vi "Convert State For Save.vi"(2 "Container State":T1, 3 "Display State":T2) -> (1 "Display State To Save":variant)   [LabVIEW 2017, in "3D Bar.xctl"]
uses:
  <vilib>/Math Plots/3D Math Plots/3D Bar/3D Bar XCtrl/3D Bar.xctl
  <vilib>/Math Plots/3D Math Plots/3D Bar/3D Bar XCtrl/State.ctl
  <vilib>/Math Plots/3D Math Plots/3D Bar/3D Bar/3D Bar.lvclass
  e:/builds/penguin/labview/branches/2017/dev/dist/vi.lib/Math Plots/3D Math Plots/3D Plot/3D Plot/3D Plot.lvclass
  <vilib>/Math Plots/3D Math Plots/3D Plot/Action String/3DMathPlot Ctrl Act Queue.ctl
  <vilib>/Math Plots/3D Math Plots/3D Plot/Action String/3DMathPlot Ctrl Act Cluster.ctl
  <vilib>/Math Plots/3D Math Plots/3D Plot/Action String/3DMathPlot State Class.ctl
  <vilib>/_xctls/Container State.ctl
  <vilib>/Math Plots/3D Math Plots/3D Plot/3D Plot/3D Plot.lvclass
  <vilib>/_xctls/XControlSupport.lvlib
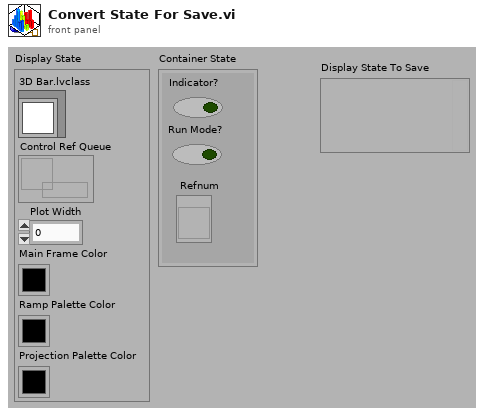
[diagram p1: front panel]
types:
  T1 = typedef "XControlSupport.lvlib/Container State.ctl" = cluster{"Indicator?":bool, "Run Mode?":bool, " Refnum":refnum<vi>}
  T2 = typedef "3D Bar.xctl/State.ctl" = cluster{"3D Bar.lvclass":refnum<class "3D Bar.lvclass">, "Control Ref Queue":T3, "Plot Width":u32, "Main Frame Color":u32, "Ramp Palette Color":u32, "Projection Palette Color":u32}
  T3 = typedef "3DMathPlot Ctrl Act Queue.ctl" = refnum<queue>
  T4 = enum32{"Towards X-Y Plane", "Towards X-Z Plane", "Towards Y-Z Plane", "User Defined"}
  T5 = typedef "3DMathPlot Ctrl Act Cluster.ctl" = cluster{"3D Picture Control":refnum<vi>, "Render Window Refnum":refnum<vi>, "XY Graph":refnum<vi>, "Intensity Graph":refnum<vi>, "Color Legend Palette":refnum<vi>, "Projection Palette":refnum<vi>, "XControl  Ref":refnum<vi>, "Facade Ref":refnum<vi>, "Export Image Ref":refnum<vi>, "Clear Data Flag":bool, "Display State Change Class":T6}
  T6 = typedef "3DMathPlot State Class.ctl" = enum16{"Update All Objects (Undo)", "Update Light Object Only", "Update Axis Object Only", "Update Plot Object Only", "Update Cursor Object Only", "Update Axis Plot Cursor Objects", "No Update"}
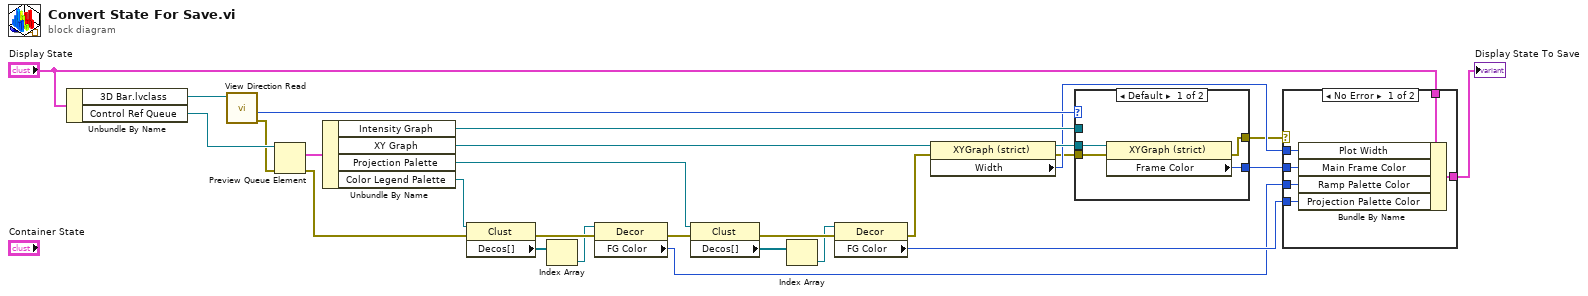
[diagram p0: block diagram]
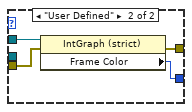
[diagram p3: hidden frame]
diagram:
  n1 = Unbundle By Name("Display State") -> ("3D Bar.lvclass"=w12:refnum<class "3D Bar.lvclass">, "Control Ref Queue"=w27:T3)
  n2 = call <vilib>:"View Direction Read.vi"("3D Plot.lvclass in"=w12) -> ("error out"=w9:errorcluster, "Value"=w11:T4)  [unwired: 8 in, 1 out]
  n3 = Preview Queue Element(queue=w27, error in (no error)=w9) -> (element=w26:T5, error out=w13:errorcluster)  [unwired: 3 out]
  n4 = Unbundle By Name(w26) -> ("Intensity Graph"=w10:refnum<vi>, "XY Graph"=w7:refnum<vi>, "Projection Palette"=w18:refnum<vi>, "Color Legend Palette"=w14:refnum<vi>)
  n5 = property class="Clust"(reference=w14, error in=w13) -> (error out=w23:errorcluster, "Decos[]"=w19:refnum<vi>[])  [unwired: 1 out]
  n6 = Index Array(array=w19) -> (element=w20:refnum<vi>)  [unwired: 1 in]
  n7 = property class="Decor"(reference=w20, error in=w23) -> (error out=w24:errorcluster, "FG Color"=w16:u32)  [unwired: 1 out]
  n8 = property class="Clust"(reference=w18, error in=w24) -> (error out=w25:errorcluster, "Decos[]"=w22:refnum<vi>[])  [unwired: 1 out]
  n9 = Index Array(array=w22) -> (element=w21:refnum<vi>)  [unwired: 1 in]
  n10 = property class="Decor"(reference=w21, error in=w25) -> (error out=w3:errorcluster, "FG Color"=w17:u32)  [unwired: 1 out]
  n11 = property class="XYGraph (strict)"(reference=w7, error in=w3) -> (reference out=w6:refnum<vi>, error out=w2:errorcluster, "Width"=w5:u32)
  n12 = case shown="Default" w11 {
    tunnel: w6 -> [w31 _]
    tunnel: [w30 w34] -> w15
    tunnel: w10 -> [_ w35]
    tunnel: w2 -> [w29 w33]
    tunnel: [w28 w32] -> w1
    frame Default {
      n13 = property class="XYGraph (strict)"(reference=w31, error in=w29) -> (error out=w28:errorcluster, "Frame Color"=w30:u32)  [unwired: 1 out]
    }
    frame "User Defined" {
      n14 = property class="IntGraph (strict)"(reference=w35, error in=w33) -> (error out=w32:errorcluster, "Frame Color"=w34:u32)  [unwired: 1 out]
    }
  }
  n15 = case shown="No Error" w1 {
    tunnel: w17 -> [w41 _]
    tunnel: w16 -> [w40 _]
    tunnel: w15 -> [w39 _]
    tunnel: "Display State" -> [w38 w42]
    tunnel: w5 -> [w37 _]
    tunnel: [w36 w42] -> w4
    frame No Error {
      n16 = Bundle By Name(cluster=w38, "Plot Width"=w37, "Main Frame Color"=w39, "Ramp Palette Color"=w40, "Projection Palette Color"=w41) -> (w36:T2)
    }
    frame Error {
    }
  }
  "Display State To Save" <- w4
